vi "AcknowledgeMessage.vi"(8 "error in (no error)":errorcluster, 9 "acknowledge":bool=TRUE, 10 "message header":T1, 11 "subscriber in":refnum<class "IcmMessageSubscriber.lvclass">) -> (0 "error out":errorcluster, 3 "subscriber out":refnum<class "IcmMessageSubscriber.lvclass">)   [LabVIEW 2017, in "IcmMessageSubscriber.lvclass"]
doc: "Acknowledges the message specified in the message header."
uses:
  <vilib>/addons/InsightCM/MessageBus/MessageSubscriber/IcmMessageSubscriber.lvclass
  <vilib>/addons/InsightCM/MessageBus/Base/controls/MessageHeader.ctl
  <vilib>/addons/InsightCM/MessageBus/Base/controls/KeyValuePair.ctl
  <vilib>/addons/InsightCM/MessageBus/MessageSubscriber/IcmMessageSubscriber.lvclass/IcmMessageSubscriber.ctl
  C:/Program Files (x86)/National Instruments/LabVIEW 2017/vi.lib/addons/InsightCM/Binaries/LabviewMessageAdapter.dll
  Binaries/LabviewMessageAdapter.dll
  <vilib>/addons/InsightCM/Utilities/PropertyHelpers/PropertyHelpers.lvlib
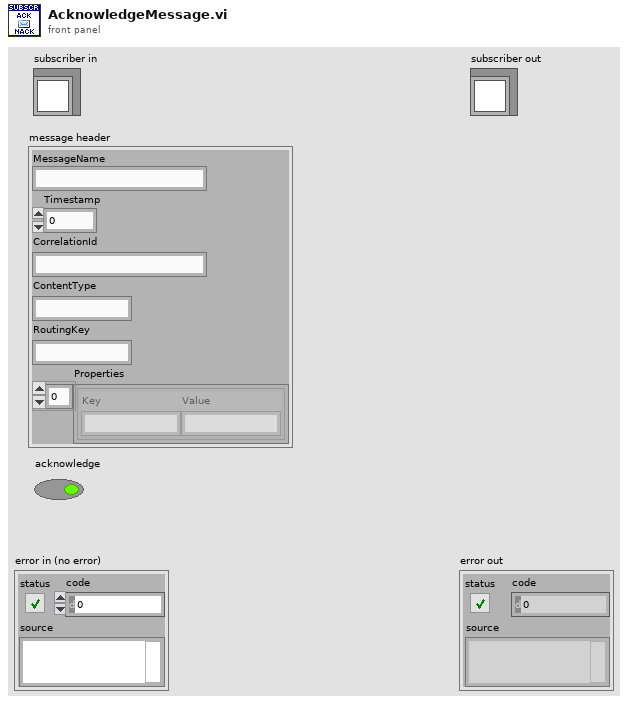
[diagram p1: front panel]
types:
  T1 = typedef "MessageHeader.ctl" = cluster{"MessageName":string, "Timestamp":i64, "CorrelationId":string, "ContentType":string, "RoutingKey":string, "Properties":T2[]}
  T2 = typedef "KeyValuePair.ctl" = cluster{"Key":string, "Value":string}
  T3 = typedef "MessageSubscriberDvr.ctl" = refnum<data-value>
  T4 = typedef "MessageSubscriberData.ctl" = cluster{"Subscriber":refnum<k24>}
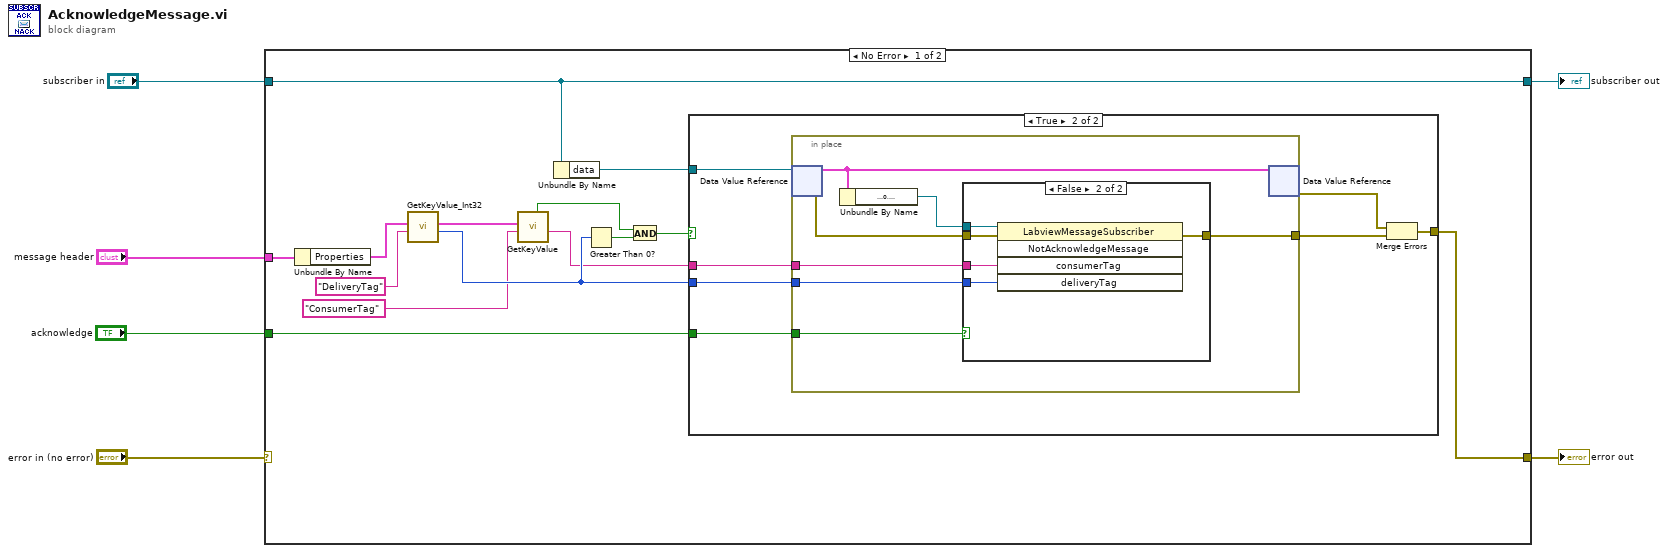
[diagram p0: block diagram]
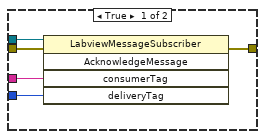
[diagram p3: hidden frame]
diagram:
  n1 = case shown="No Error" "error in (no error)" {
    selector: "error in (no error)" -> [_ w46]
    tunnel: [w19 w46] -> w5
    tunnel: "subscriber in" -> [w18 w45]
    tunnel: [w18 w45] -> w3
    tunnel: "acknowledge" -> [w17 _]
    tunnel: "message header" -> [w16 _]
    frame No Error {
      n2 = Unbundle By Name(w16) -> ("Properties"=w13:T2[])
      n3 = call <vilib>:"GetKeyValue_Int32.vi"("key"="DeliveryTag" ("Key"), "key value pairs"=w13) -> ("value"=w10:i32, "key value pairs out"=w12:T2[])  [unwired: 7 in, 1 out]
      n4 = call <vilib>:"GetKeyValue.vi"("key"="ConsumerTag" ("Key"), "key value pairs"=w12) -> ("value"=w8:string, "found"=w7:bool)  [unwired: 7 in, 1 out]
      n5 = Unbundle By Name(w18) -> ("data"=w20:T3)
      n6 = Greater Than 0?(x=w10) -> (x > 0?=w15:bool)
      n7 = And(x=w7, y=w15) -> (x .and. y?=w14:bool)
      n8 = case shown="True" w14 {
        tunnel: w20 -> [_ w27]
        tunnel: w8 -> [_ w24]
        tunnel: [_ w23] -> w19
        tunnel: w17 -> [_ w22]
        tunnel: w10 -> [_ w21]
        frame False {
        }
        frame True {
          n9 = in-place {
            in-place-border: [w33] -> w25
            in-place-border: w24 -> [w30]
            in-place-border: w22 -> [w28]
            in-place-border: w21 -> [w29]
            n10 = in-place-dvr #1(w27) -> (w34:T4, w32:errorcluster)
            n11 = Unbundle By Name(w34) -> ("Subscriber"=w31:refnum<k24>)
            n12 = case shown="False" w28 {
              tunnel: [w39 w44] -> w33
              tunnel: w32 -> [w38 w43]
              tunnel: w31 -> [w37 w42]
              tunnel: w30 -> [w36 w41]
              tunnel: w29 -> [w35 w40]
              frame True {
                n13 = invoke class="LabviewMessageSubscriber" method="AcknowledgeMessage"(reference=w37, error in=w38, "consumerTag"=w36, "deliveryTag"=w35) -> (error out=w39:errorcluster)  [unwired: 1 in, 4 out]
              }
              frame False {
                n14 = invoke class="LabviewMessageSubscriber" method="NotAcknowledgeMessage"(reference=w42, error in=w43, "consumerTag"=w41, "deliveryTag"=w40) -> (error out=w44:errorcluster)  [unwired: 1 in, 4 out]
              }
            }
            n15 = in-place-dvr #1(w34) -> (w26:errorcluster)  [unwired: 1 out]
          }
          n16 = Merge Errors(w26, w25) -> (w23:errorcluster)
        }
      }
    }
    frame Error {
    }
  }
  "error out" <- w5
  "subscriber out" <- w3
